vi "Get_SLOPE_data_from_file 2016.vi"(11 "Slopes File Path":path=path "D:/Cascade/Data/Output Files/slopes.txt") -> (0 "Last_Pressure_Slope":dbl format="%.2f", 1 "Last_Flow_Slope":dbl format="%.2f", 2 "Last_String_Pot_Slope":dbl format="%.2f", 3 "Output_array":sgl[][](array[numeric]) format="%.2f")   [LabVIEW 2016]
uses:
  <vilib>/Utility/file.llb/Read Delimited Spreadsheet (DBL).vi
panel:
  out "file or folder exists?":bool
  out "error out":errorcluster
  out "Last_KPRO_Box_Number":dbl
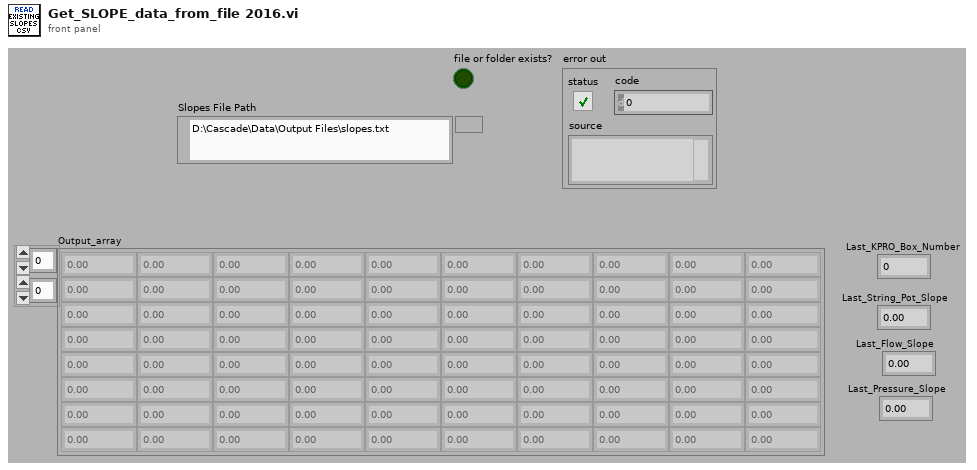
[diagram p1: front panel]
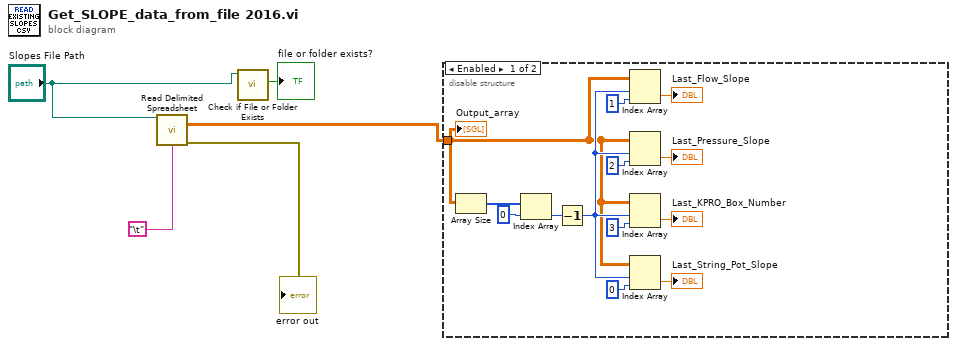
[diagram p0: block diagram]
diagram:
  n1 = call-poly <vilib>:"Read Delimited Spreadsheet.vi"("file path (dialog if empty)"="Slopes File Path", "delimiter (\\t)"="\t") -> ("all rows"=w3:dbl[][], "error out"=→"error out":errorcluster)  [unwired: 8 in, 4 out]
  n2 = call <vilib>:"Check if File or Folder Exists.vi"("path"="Slopes File Path") -> ("file or folder exists?"=→"file or folder exists?":bool)  [unwired: 8 in, 2 out]
  n3 = disable-structure shown="Enabled" {
    disable-tunnel: w3 -> [w6 _]
    frame Enabled {
      n4 = Array Size(array=w6) -> (size(s)=w17:i32[])
      n5 = Index Array(array=w17, index=0) -> (element=w16:i32)
      n6 = Decrement(x=w16) -> (x-1=w9:i32)
      n7 = Index Array(array=w6, index (row)=w9, index (col)=1 ("disabled index (col)")) -> (element=→"Last_Flow_Slope":dbl)
      n8 = Index Array(array=w6, index (row)=w9, index (col)=2 ("index")) -> (element=→"Last_Pressure_Slope":dbl)
      n9 = Index Array(array=w6, index (row)=w9, index (col)=3 ("index")) -> (element=→"Last_KPRO_Box_Number":dbl)
      n10 = Index Array(array=w6, index (row)=w9, index (col)=0 ("index")) -> (element=→"Last_String_Pot_Slope":dbl)
      "Output_array" <- w6
    }
    frame Disabled {
    }
  }
